vi "Write Project Refnum.vi"(8 "error in (no error)":errorcluster, 10 "Project Refnum":refnum<vi>, 11 "Test Runner.Project in":refnum<class "Test Runner.Project.lvclass">) -> (0 "error out":errorcluster, 3 "Test Runner.Project out":refnum<class "Test Runner.Project.lvclass">)   [LabVIEW 2013, in "Caraya.lvlib" / "Test Runner.Project.lvclass"]
uses:
  Test Runner.Project.lvclass
  Test Runner.Project.lvclass/Test Runner.Project.ctl
  Test Runner/Test Runner.lvclass
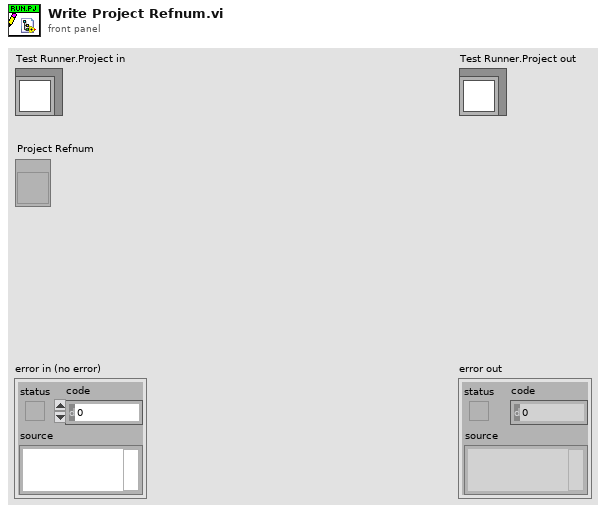
[diagram p1: front panel]
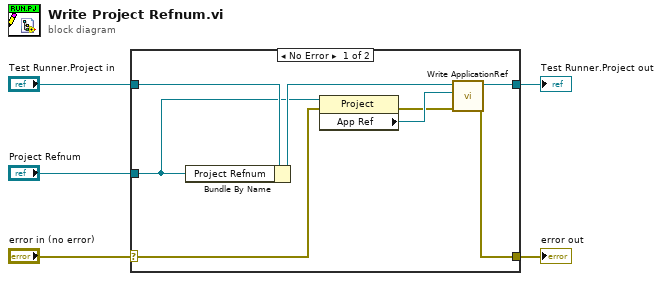
[diagram p0: block diagram]
diagram:
  n1 = case shown="No Error" "error in (no error)" {
    selector: "error in (no error)" -> [w7 w14]
    tunnel: [w6 w14] -> w4
    tunnel: [w11 w15] -> w2
    tunnel: "Test Runner.Project in" -> [w13 w15]
    tunnel: "Project Refnum" -> [w10 _]
    frame No Error {
      n2 = Bundle By Name(cluster=w13, "Project Refnum"=w10) -> (w12:refnum<class "Test Runner.Project.lvclass">)
      n3 = property class="Project"(reference=w10, error in=w7) -> (error out=w8:errorcluster, "App Ref"=w9:refnum<vi>)  [unwired: 1 out]
      n4 = call "Write ApplicationRef.vi"("error in (no error)"=w8, "Application"=w9, "Test Runner in"=w12) -> ("error out"=w6:errorcluster, "Test Runner out"=w11:refnum<class "Test Runner.Project.lvclass">)  [unwired: 7 in]
    }
    frame Error {
    }
  }
  "error out" <- w4
  "Test Runner.Project out" <- w2
